vi "movePI2.vi"(2 "PI Stage Error":errorcluster, 3 "move to position":dbl=0.00015 format="%.5f") -> (0 "final position":dbl, 1 "PI Stage Error 2":errorcluster)   [LabVIEW 2014]
panel:
  out "Position":dbl[](array[numeric]) format="%.6f"
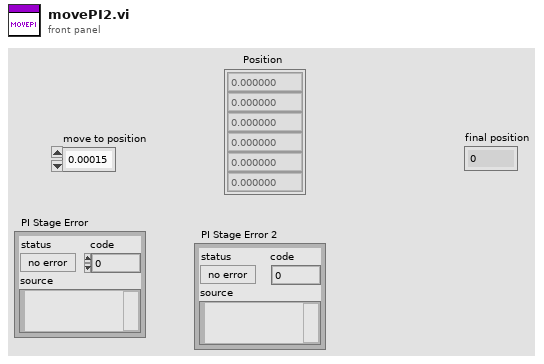
[diagram p1: front panel]
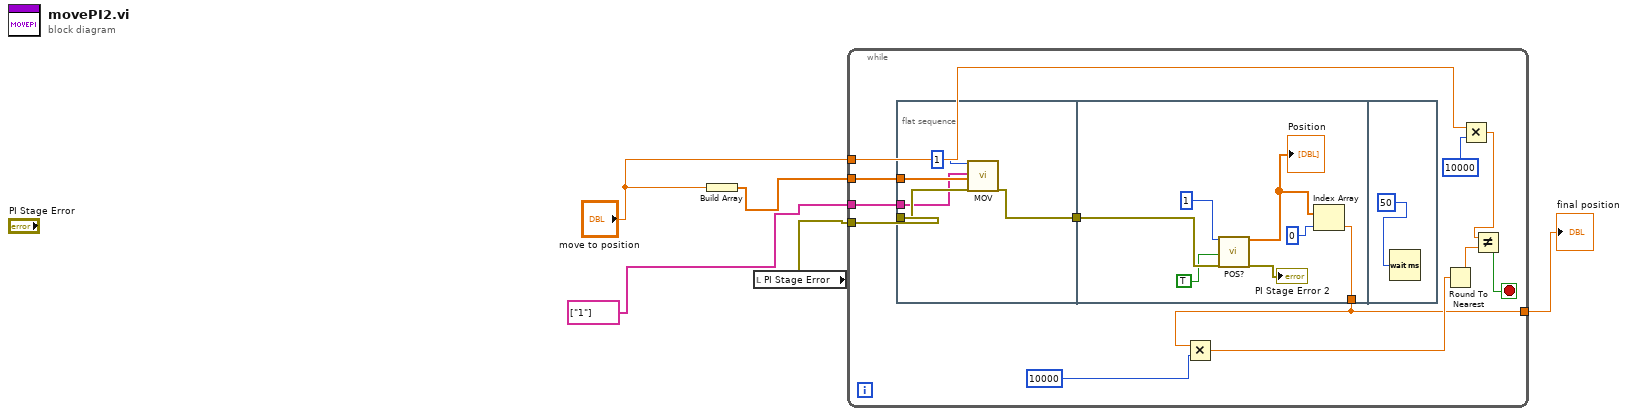
[diagram p0: block diagram]
diagram:
  n1 = Build Array("move to position") -> (w2:dbl[])
  n2 = local read "PI Stage Error"() -> (w3:errorcluster)
  n3 = while {
    tunnel: "move to position" -> [w14]
    tunnel: w3 -> [w16]
    tunnel: [w9] -> w4
    tunnel: w2 -> [w7]
    tunnel: string[] ["1"] ("Conn. Axes") -> [w6]
    stop <- w17 stop-if-true
    n4 = flat-sequence {
      tunnel: w16 -> [w22]
      tunnel: [w21] -> w8
      tunnel: w7 -> [w19]
      tunnel: w6 -> [w18]
      tunnel: [w23] -> w9
      tunnel: w8 -> [w29]
      frame #0 {
        n5 = call "MOV.vi"("System no."=1, "Axes to move"=w18, "Position values"=w19, "error in"=w22) -> ("error out"=w21:errorcluster)  [unwired: 15 in]
      }
      frame #1 {
        n6 = call "POS?.vi"("System no."=1, "All axes?"=TRUE, "error in"=w29) -> ("Position"=w25:dbl[], "error out"=→"PI Stage Error 2":errorcluster)  [unwired: 15 in]
        "Position" <- w25
        n7 = Index Array(array=w25, index=0) -> (element=w23:dbl)
      }
      frame #2 {
        n8 = Wait (ms)(milliseconds to wait=50) -> ()  [unwired: 1 out]
      }
    }
    n9 = Multiply(x=w9, y=10000 ("System no.")) -> (x*y=w10:dbl)
    n10 = Round To Nearest(number=w10) -> (nearest integer value=w15:dbl)
    n11 = Multiply(x=w14, y=10000 ("System no.")) -> (x*y=w12:dbl)
    n12 = Not Equal?(x=w12, y=w15) -> (x != y?=w17:bool)
  }
  "final position" <- w4
